vi "TTA_MATLAB_RxOutputPowerTest.vi"(0 "Sub-Function Name":string, 1 "Instrument Cluster In":T2, 5 "Test Group":string, 11 "error in":errorcluster) -> (4 "RxOutput\nPower Results":T1(array[cluster]), 6 "SubTestSuccess":dbl[](array[numeric]), 12 "Instrument Cluster Out":T2, 15 "error out":errorcluster)   [LabVIEW 2016]
uses:
  TTA_Controls/TTA_Control_Complete_Settings_Cluster.ctl
  TTA_Controls/TTA_Control_Instrument_Cluster.ctl
  TTA_Globals/TTA_Global_Complete_Settings.vi
panel:
  out "Channel":string
  out "Rx":string
  out "Test Status":string
  in  "Complete Settings Cluster":T3
  out "RFICs":i32[](array[numeric])
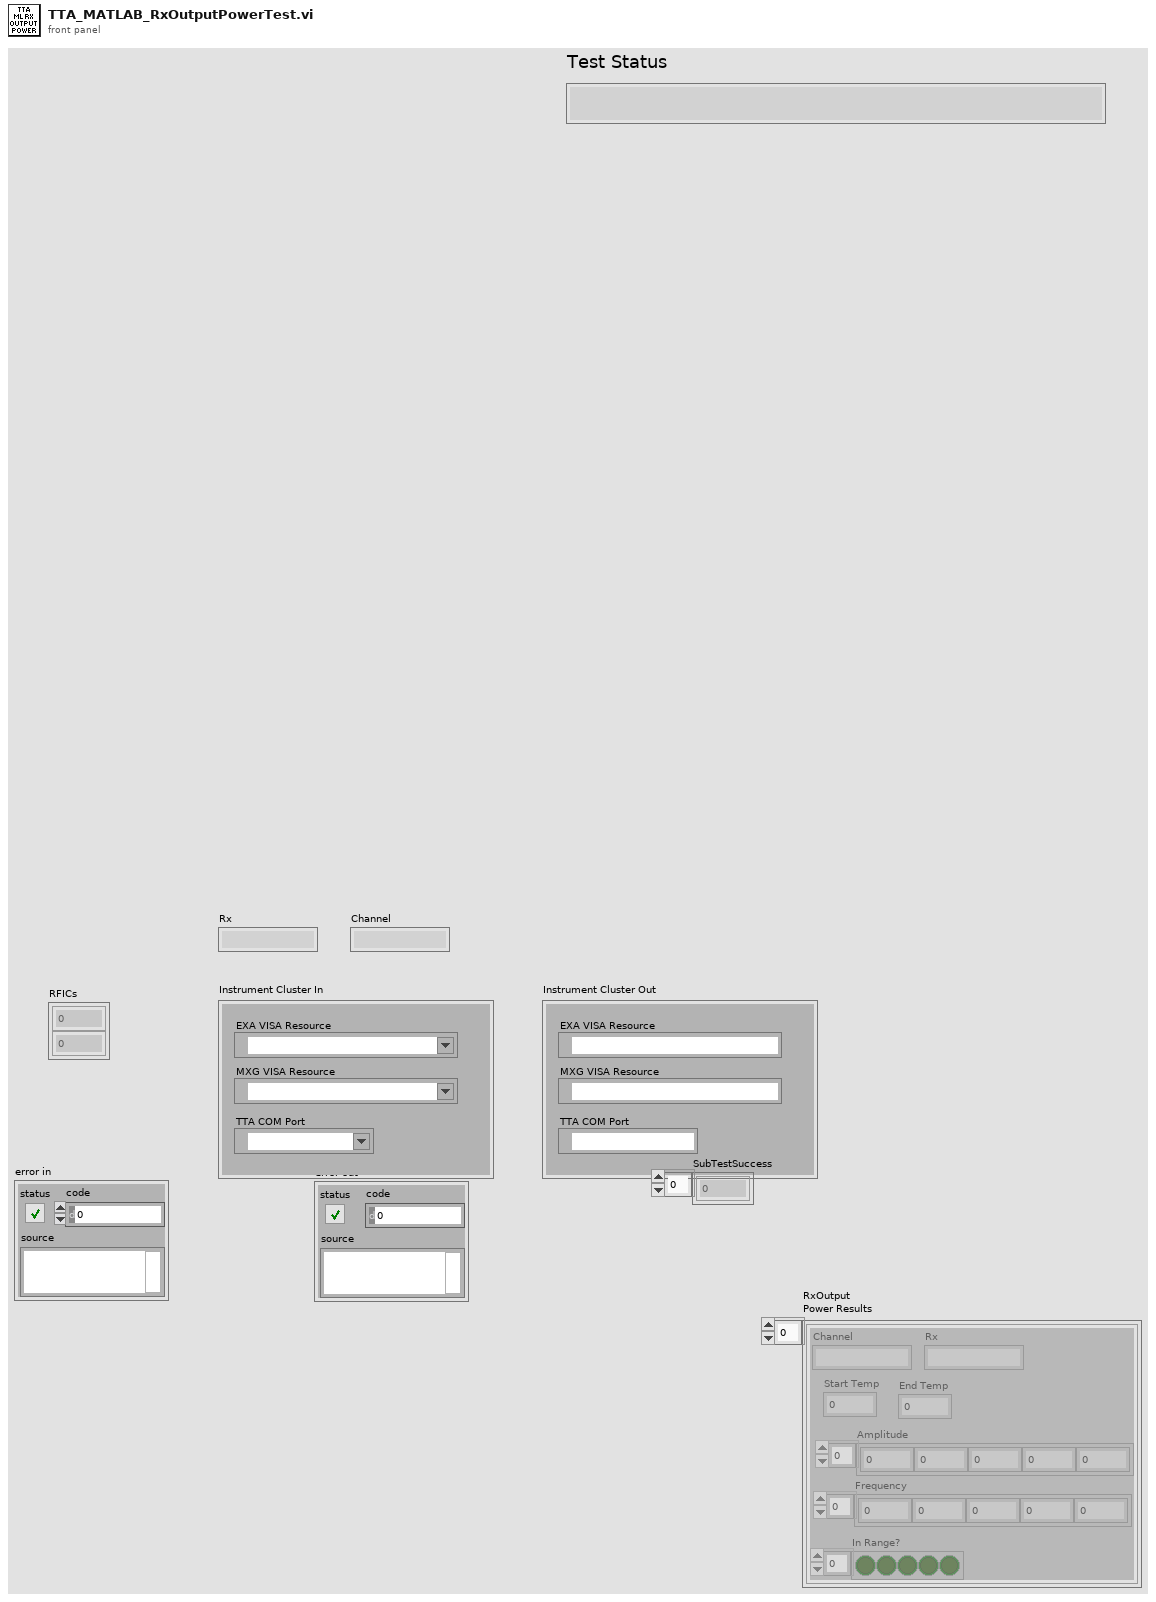
[diagram p1: front panel]
types:
  T1 = cluster{"Channel":string, "Rx":string, "Start Temp":dbl, "End Temp":dbl, "Amplitude":dbl[], "Frequency":dbl[], "In Range?":bool[]}[]
  T2 = typedef "TTA_Control_Instrument_Cluster.ctl" = cluster{"EXA VISA Resource":refnum<visa-resource-name>, "MXG VISA Resource":refnum<visa-resource-name>, "TTA COM Port":refnum<visa-resource-name>}
  T3 = typedef "TTA_Control_Complete_Settings_Cluster.ctl" = cluster{"Brief Cluster":cluster{"STM Firmware File":string, "STM Firmware Address":string, "Required SW Version":string, "Template Used":string}, "Instrument Setting Cluster":cluster{"BDSFreq":dbl, "BDS Amp":dbl, "TxRFCal_Freq":dbl, "TxRFCal_Amp":dbl, "RxRFCal_Freq":dbl, "RxRFCal_Freq":dbl, "TxIF_Freq":dbl, "TxIF_Amp":dbl, "Tx_Output_Power_Signal_Freq":dbl, "Tx_ACPR_Signal_Freq":dbl, "Rx_RF_Freq":dbl, "Rx_RF_Amp":dbl, "Rx_Output_Power_Signal_Freq":dbl, "Rx_Output_Power_Sense_Freq":dbl}, "PAL Calibration\nInputs Cluster":cluster{"Amplitude Range\nMax(dBm)":dbl, "Amplitude Range\nMin(dBm)":dbl, "Amplitude Least\nCriteria (dBm)":dbl, "Frequency 1":dbl, "Frequency 2":dbl, "Frequency 3":dbl, "CAL Amplitude\nDecrement (dB)":dbl, "CAL Amplitude\nIncrement(dB)":dbl, "DownloadFile":string}, "TxOffset Cal Cluster":cluster{"Tx1 Offset (dB)":dbl, "Tx2 Offset (dB)":dbl, "Tx3 Offset (dB)":dbl, "Tx4 Offset (dB)":dbl, "Total RF Tx Loss (dB)":dbl}, "RxOffset Cal Cluster":cluster{"Rx1 Offset (dB)":dbl, "Rx2 Offset (dB)":dbl, "Rx3 Offset (dB)":dbl, "Rx4 Offset (dB)":dbl, "Total RF Rx Loss (dB)":dbl}, "TX Output Power Settings Cluster":cluster{"Frequency Sweep (MHz)":dbl[], "Sig Gen \nPower (dBm)":dbl, "Span (kHz)":dbl, "RBW (Hz)":dbl, "Ref Level (dBm)":dbl, "Low Power \nLimit":dbl, "High Power \nLimit":dbl, "DigAtt Max":dbl, "DigAtt Min":dbl}, "Tx ACPR Settings Cluster":cluster{"ACPR Filename":string, "Sampling Rate":dbl, "Power (dBm)":dbl, "IF Frequency Sweep (MHz)":dbl[], "State Name":string, "Mechanical\nAttenuation":dbl, "RefLevel Offset":dbl, "Amplitude Range\nMax (dBm)":dbl, "Amplitude Range\nMin (dBm)":dbl, "Cal Amp \nIncrement (dB)":dbl, "Cal Amp\nDecrement (dB)":dbl}, "Power Cal Cluster":cluster{"Power List (dBm)":dbl[], "Frequency (MHz)":dbl[], "Cal Decrement (dB)":dbl, "Cal Increment (dB)":dbl}, "Rx Received Power Settings Cluster":cluster{"Frequency Sweep (MHz)":dbl[], "Power (dBm)":dbl, "Span (kHz)":dbl, "RBW (Hz)":dbl, "Ref Level":dbl, "Low Power \nLimit (dBm)":dbl, "High Power\nLimit (dBm)":dbl}, "Tx Output Power Criteria Cluster":cluster{"CH1-TX1 \nMin":dbl, "CH1-TX1\nMax":dbl, "CH1-TXx3\nMin ":dbl, "CH1-TXx3\nMax":dbl, "CH2-TX1\nMin":dbl, "CH2-TX1\nMax":dbl, "CH2-TXx3\nMin":dbl, "CH2-TXx3\nMax":dbl}, "Tx ACPR Criteria Cluster":cluster{"Min Inband":dbl, "Max Close Outband":dbl, "Max Far Outband":dbl}, "Rx Output Power Criteria Cluster":cluster{"CH1-RX1 \nMin":dbl, "CH1-RX1 \nMax":dbl, "CH1-RXx3 \nMin":dbl, "CH1-RXx3\nMax":dbl, "CH2-RX1\nMin":dbl, "CH2-RX1\nMax":dbl, "CH2-RXx3\nMin":dbl, "CH2-RXx3\nMax":dbl}}
  T4 = cluster{"BDSFreq":dbl, "BDS Amp":dbl, "TxRFCal_Freq":dbl, "TxRFCal_Amp":dbl, "RxRFCal_Freq":dbl, "RxRFCal_Freq":dbl, "TxIF_Freq":dbl, "TxIF_Amp":dbl, "Tx_Output_Power_Signal_Freq":dbl, "Tx_ACPR_Signal_Freq":dbl, "Rx_RF_Freq":dbl, "Rx_RF_Amp":dbl, "Rx_Output_Power_Signal_Freq":dbl, "Rx_Output_Power_Sense_Freq":dbl}
  T5 = cluster{"Frequency Sweep (MHz)":dbl[], "Power (dBm)":dbl, "Span (kHz)":dbl, "RBW (Hz)":dbl, "Ref Level":dbl, "Low Power \nLimit (dBm)":dbl, "High Power\nLimit (dBm)":dbl}
  T6 = cluster{"Channel":string, "Rx":string, "Start Temp":dbl, "End Temp":dbl, "Amplitude":dbl[], "Frequency":dbl[], "In Range?":bool[]}
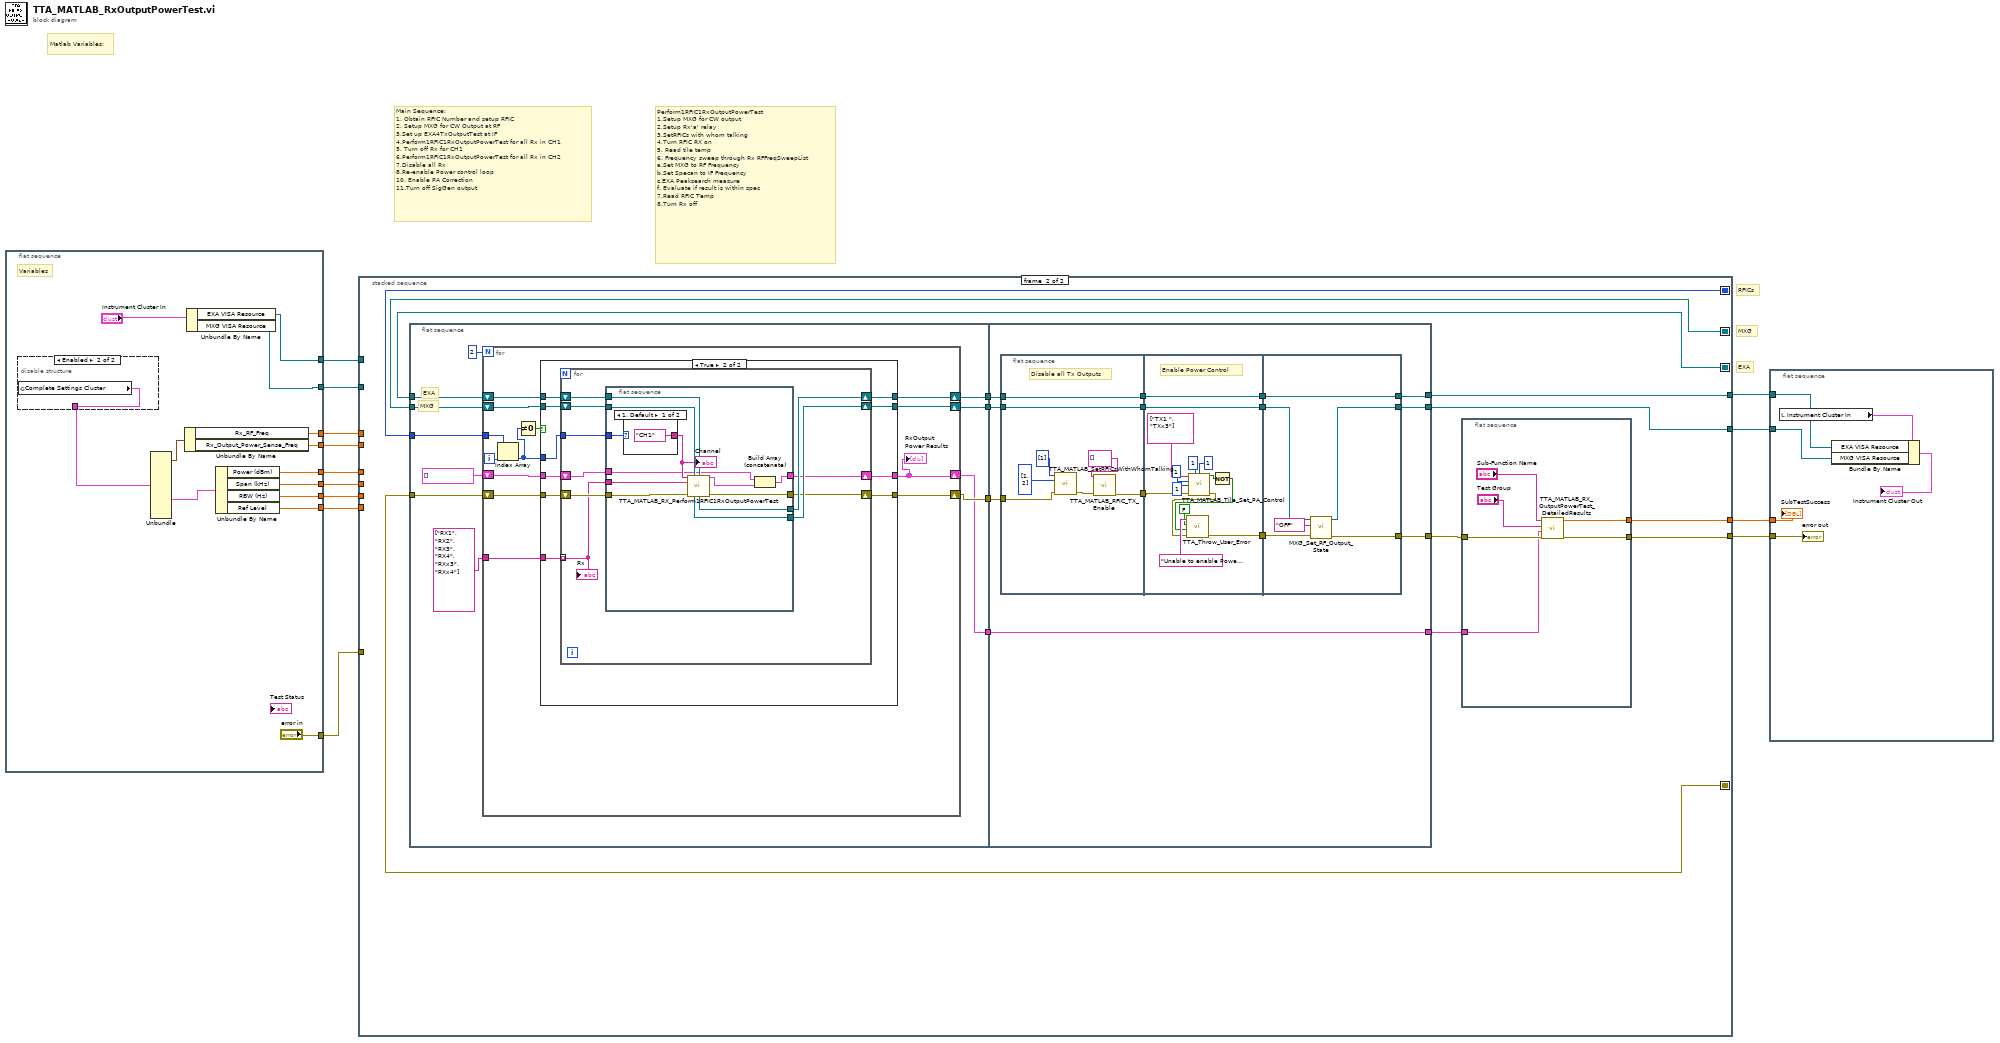
[diagram p0: block diagram]
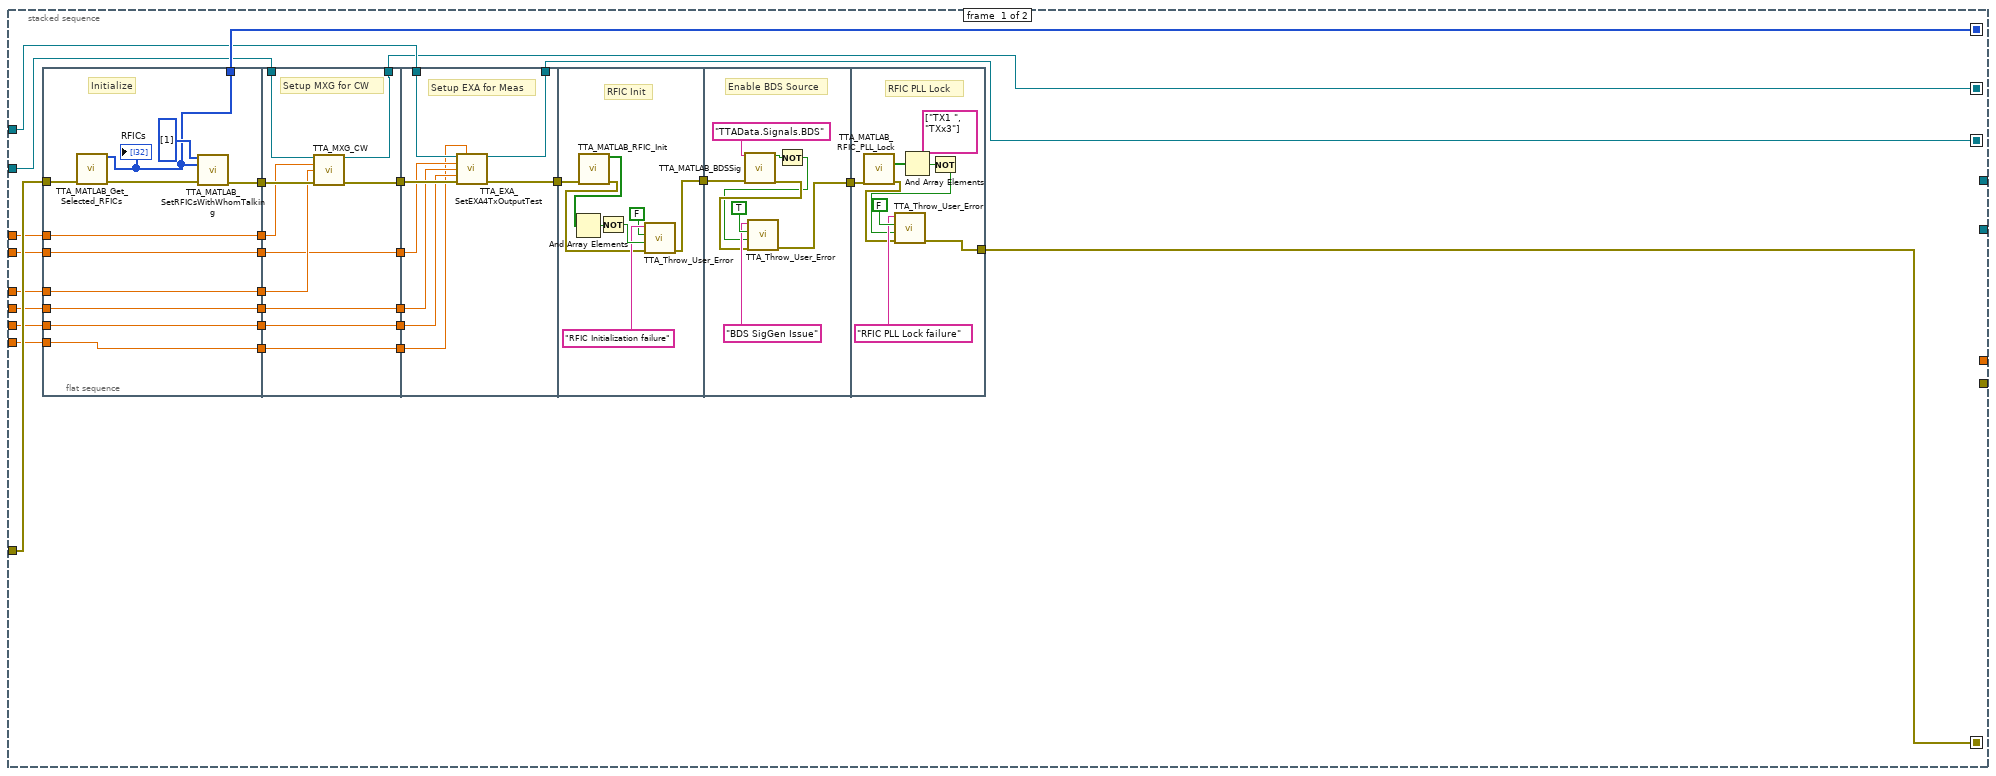
[diagram p2: hidden frame]
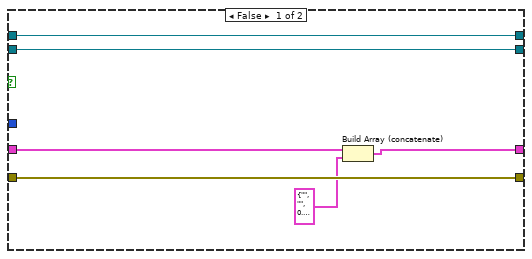
[diagram p3: hidden frame]
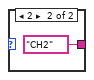
[diagram p4: hidden frame]
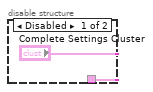
[diagram p5: hidden frame]
diagram:
  # "RFICs"
  # "EXA"
  # "MXG"
  # "Matlab Variables:"
  # "Main Sequence:\n1. Obtain RFIC Number and setup RFIC\n2. Setup MXG for CW Output at RF\n3.Set up EXA4TxOutputTest at IF\n4.Perform1RFIC1RxOutputPowerTest for all Rx in CH1\n5. Turn off Rx for CH1\n6.Perform1RFIC1RxOutputPowerTest for all Rx in CH2\n7.Disable all Rx\n8.Re-enable Power control loop\n10. Enable PA Correction\n11.Turn off SigGen output"
  # "Perform1RFIC1RxOutputPowerTest\n1.Setup MXG for CW output\n2.Setup Rx'a' relay\n3.SetRFICs with whom talking\n4.Turn RFIC RX on\n5. Read tile temp\n6. Frequency sweep through Rx RFFreqSweepList\na.Set MXG to RF Frequency\nb.Set Specan to IF Frequency\nc.EXA Peaksearch measure\nf. Evaluate if result is within spec\n7.Read RFIC Temp\n8.Turn Rx off"
  n1 = flat-sequence {
    tunnel: ["error in"] -> w13
    tunnel: [w23] -> w12
    tunnel: [w22] -> w11
    tunnel: [w19] -> w7
    tunnel: [w18] -> w6
    tunnel: [w17] -> w5
    tunnel: [w16] -> w4
    tunnel: [w15] -> w3
    tunnel: [w14] -> w2
    frame #0 {
      # "Variables"
      n2 = disable-structure shown="Enabled" {
        disable-tunnel: ["Complete Settings Cluster" w28] -> w26
        frame Disabled {
        }
        frame Enabled {
          n3 = global read "TTA_Global_Complete_Settings.vi" "Complete Settings Cluster"() -> (w28:T3)
        }
      }
      n4 = Unbundle(w26) -> ("Instrument Setting Cluster"=w20:T4, "Rx Received Power Settings Cluster"=w21:T5)  [unwired: 10 out]
      n5 = Unbundle By Name(w20) -> ("Rx_RF_Freq"=w19:dbl, "Rx_Output_Power_Sense_Freq"=w17:dbl)
      n6 = Unbundle By Name("Instrument Cluster In") -> ("EXA VISA Resource"=w23:refnum<visa-resource-name>, "MXG VISA Resource"=w22:refnum<visa-resource-name>)
      n7 = Unbundle By Name(w21) -> ("Power (dBm)"=w18:dbl, "Span (kHz)"=w16:dbl, "RBW (Hz)"=w15:dbl, "Ref Level"=w14:dbl)
    }
  }
  n8 = stacked-sequence {
    seq-local: [w55 _] -> [_ w123]
    seq-local: [w31 _] -> [_ w121]
    seq-local: [w29 _] -> [_ w122]
    seq-local: [w30 _] -> [_ w120]
    tunnel: w13 -> [w56 _]
    tunnel: w12 -> [w44 _]
    tunnel: w11 -> [w51 _]
    tunnel: [_ w111] -> w10
    tunnel: [_ w116] -> w9
    tunnel: [_ w115] -> w8
    tunnel: w7 -> [w50 _]
    tunnel: w6 -> [w48 _]
    tunnel: w5 -> [w43 _]
    tunnel: w4 -> [w40 _]
    tunnel: w3 -> [w39 _]
    tunnel: w2 -> [w38 _]
    tunnel: [_ w110] -> w1
    frame #0 {
      n9 = flat-sequence {
        tunnel: w56 -> [w65]
        tunnel: [w64] -> w55
        tunnel: [w63] -> w54
        tunnel: w50 -> [w62]
        tunnel: [w62] -> w49
        tunnel: w48 -> [w61]
        tunnel: [w61] -> w47
        tunnel: w43 -> [w60]
        tunnel: [w60] -> w41
        tunnel: w40 -> [w59]
        tunnel: w39 -> [w58]
        tunnel: w38 -> [w57]
        tunnel: [w59] -> w36
        tunnel: [w58] -> w34
        tunnel: [w57] -> w32
        tunnel: w54 -> [w76]
        tunnel: [w73] -> w46
        tunnel: w51 -> [w77]
        tunnel: w49 -> [w75]
        tunnel: w47 -> [w74]
        tunnel: [w72] -> w42
        tunnel: w41 -> [w72]
        tunnel: [w71] -> w37
        tunnel: w36 -> [w71]
        tunnel: [w70] -> w35
        tunnel: w34 -> [w70]
        tunnel: [w69] -> w33
        tunnel: w32 -> [w69]
        tunnel: [w68] -> w30
        tunnel: w46 -> [w85]
        tunnel: [w78] -> w45
        tunnel: w44 -> [w84]
        tunnel: w42 -> [w83]
        tunnel: w37 -> [w82]
        tunnel: w35 -> [w81]
        tunnel: w33 -> [w80]
        tunnel: [w79] -> w29
        tunnel: w45 -> [w88]
        tunnel: [w86] -> w53
        tunnel: w53 -> [w97]
        tunnel: [w95] -> w52
        tunnel: w52 -> [w104]
        tunnel: [w102] -> w31
        frame #0 {
          # "Initialize"
          n10 = call "TTA_MATLAB_Get_Selected_RFICs.vi"("error in"=w65) -> ("RFICs"=w64:i32[], "error out"=w66:errorcluster)  [unwired: 13 in]
          "RFICs" <- w64
          n11 = call "TTA_MATLAB_SetRFICsWithWhomTalking.vi"("Panel Array"=i32[] [1], "RFIC Array"=w64, "error in"=w66) -> ("error out"=w63:errorcluster)  [unwired: 12 in]
        }
        frame #1 {
          # "Setup MXG for CW"
          n12 = call "TTA_MXG_CW.vi"("VISA resource In"=w77, "Frequency (MHz)"=w75, "Output Power\nLevel (dBm)"=w74, "error in"=w76) -> ("VISA resource Out"=w68:refnum<visa-resource-name>, "error out"=w73:errorcluster)  [unwired: 10 in]
        }
        frame #2 {
          # "Setup EXA for Meas"
          n13 = call "TTA_EXA_SetEXA4TxOutputTest.vi"("VISA resource In"=w84, "Reference Level (dBm)"=w80, "Frequency (MHz)"=w83, "Span (kHz)"=w82, "RBW (Hz)"=w81, "error in"=w85) -> ("VISA resource Out"=w79:refnum<visa-resource-name>, "error out"=w78:errorcluster)  [unwired: 8 in]
        }
        frame #3 {
          # "RFIC Init"
          n14 = call "TTA_MATLAB_RFIC_Init.vi"("error in"=w88) -> ("SuccessComm"=w93:bool[], "error out"=w87:errorcluster)  [unwired: 13 in]
          n15 = And Array Elements(Boolean array=w93) -> (logical AND=w92:bool)
          n16 = Not(x=w92) -> (.not. x?=w91:bool)
          n17 = call "TTA_Throw_User_Error.vi"("error in"=w87, "Error?"=w91, "Stop Execution on Fail"=FALSE, "Error Message"="RFIC Initialization failure") -> ("error out"=w86:errorcluster)  [unwired: 7 in]
        }
        frame #4 {
          # "Enable BDS Source"
          n18 = call "TTA_MATLAB_BDSSig.vi"("Signal Settings"="TTAData.Signals.BDS", "error in"=w97) -> ("Success"=w98:bool, "error out"=w96:errorcluster)  [unwired: 12 in]
          n19 = Not(x=w98) -> (.not. x?=w94:bool)
          n20 = call "TTA_Throw_User_Error.vi"("error in"=w96, "Error?"=w94, "Stop Execution on Fail"=TRUE, "Error Message"="BDS SigGen Issue") -> ("error out"=w95:errorcluster)  [unwired: 7 in]
        }
        frame #5 {
          (unwired) string[] ["TX1 ", "TXx3"] ("Channels")
          # "RFIC PLL Lock"
          n21 = call "TTA_MATLAB_RFIC_PLL_Lock.vi"("error in"=w104) -> ("SuccessComm"=w109:bool[], "error out"=w103:errorcluster)  [unwired: 11 in, 2 out]
          n22 = And Array Elements(Boolean array=w109) -> (logical AND=w106:bool)
          n23 = Not(x=w106) -> (.not. x?=w105:bool)
          n24 = call "TTA_Throw_User_Error.vi"("error in"=w103, "Error?"=w105, "Stop Execution on Fail"=FALSE, "Error Message"="RFIC PLL Lock failure") -> ("error out"=w102:errorcluster)  [unwired: 7 in]
        }
      }
    }
    frame #1 {
      n25 = flat-sequence {
        tunnel: w123 -> [w140]
        tunnel: w122 -> [w139]
        tunnel: w120 -> [w138]
        tunnel: w121 -> [w137]
        tunnel: [w136] -> w119
        tunnel: [w135] -> w118
        tunnel: [w134] -> w117
        tunnel: [w130] -> w113
        tunnel: w119 -> [w206]
        tunnel: w118 -> [w205]
        tunnel: w117 -> [w204]
        tunnel: [w197] -> w114
        tunnel: [w196] -> w116
        tunnel: [w195] -> w115
        tunnel: w113 -> [w194]
        tunnel: [w194] -> w112
        frame #0 {
          # "EXA"
          # "MXG"
          n26 = for {
            N: 2 -> [_]
            tunnel: w140 -> [w145]
            shift-right: [w151] -> w135
            shift-left: w139 -> [w150]
            shift-right: [w148] -> w134
            shift-left: w138 -> [w149]
            shift-right: [w147] -> w136
            shift-left: w137 -> [w153]
            tunnel: string[] ["RX1", "RX2", "RX3", "RX4", "RXx3", "RXx4"] -> [w152]
            shift-right: [w141] -> w130
            shift-left: T1 [] -> [w146]
            i -> [w144]
            n27 = Index Array(array=w145, index=w144) -> (element=w142:i32)
            n28 = Not Equal To 0?(x=w142) -> (x != 0?=w143:bool)
            n29 = case shown="True" w143 {
              tunnel: w153 -> [w159 w169]
              tunnel: w152 -> [_ w168]
              tunnel: [w155 w167] -> w151
              tunnel: w150 -> [w155 w166]
              tunnel: w149 -> [w154 w165]
              tunnel: [w154 w164] -> w148
              tunnel: [w159 w163] -> w147
              tunnel: w146 -> [w157 w162]
              tunnel: [w156 w161] -> w141
              tunnel: w142 -> [_ w160]
              frame False {
                n30 = Build Array (concatenate)(w157, T6 {"Channel"="", "Rx"="", "Start Temp"=0.0, "End Temp"=0.0, "Amplitude"=[], "Frequency"=[], "In Range?"=[]} ("Output Power\nResults")) -> (w156:T1)
              }
              frame True {
                n31 = for {
                  tunnel: w160 -> [w179]
                  tunnel: w168 -> [w177] mode=indexing
                  shift-right: [w176] -> w167
                  shift-left: w166 -> [w175]
                  shift-right: [w174] -> w164
                  shift-left: w165 -> [w173]
                  shift-right: [w172] -> w163
                  shift-left: w169 -> [w178]
                  shift-right: [w171] -> w161
                  shift-left: w162 -> [w170]
                  n32 = flat-sequence {
                    tunnel: w179 -> [w191]
                    tunnel: w175 -> [w190]
                    tunnel: w173 -> [w189]
                    tunnel: w178 -> [w188]
                    tunnel: w177 -> [w180]
                    tunnel: [w186] -> w176
                    tunnel: [w185] -> w174
                    tunnel: [w184] -> w172
                    tunnel: [w182] -> w171
                    tunnel: w170 -> [w181]
                    frame #0 {
                      n33 = case shown="1, Default" w191 {
                        tunnel: ["CH1" ("Channel") "CH2" ("Channel")] -> w187
                        frame 1, Default {
                        }
                        frame 2 {
                        }
                      }
                      "Channel" <- w187
                      n34 = call "TTA_MATLAB_RX_Perform1RFIC1RxOutputPowerTest.vi"("Channel"=w187, "MXG VISA Resource In"=w189, "EXA VISA Resource"=w190, "Rx"=w180, "error in"=w188) -> ("Output Power\nResults"=w183:T6, "MXG VISA Resource Out"=w185:refnum<visa-resource-name>, "EXA VISA Resource Out"=w186:refnum<visa-resource-name>, "error out"=w184:errorcluster)  [unwired: 7 in]
                      n35 = Build Array (concatenate)(w181, w183) -> (w182:T1)
                    }
                  }
                  "Rx" <- w177
                }
              }
            }
            "RxOutput\nPower Results" <- w141
          }
        }
        frame #1 {
          n36 = flat-sequence {
            tunnel: w206 -> [w212]
            tunnel: w205 -> [w208]
            tunnel: w204 -> [w207]
            tunnel: [w209] -> w203
            tunnel: [w208] -> w202
            tunnel: [w207] -> w201
            tunnel: w203 -> [w217]
            tunnel: w202 -> [w228]
            tunnel: w201 -> [w227]
            tunnel: [w228] -> w200
            tunnel: [w227] -> w199
            tunnel: [w215] -> w198
            tunnel: [w231] -> w196
            tunnel: [w234] -> w195
            tunnel: w200 -> [w234]
            tunnel: w199 -> [w232]
            tunnel: w198 -> [w233]
            tunnel: [w229] -> w197
            frame #0 {
              # "Disable all Tx Outputs"
              n37 = call "TTA_MATLAB_SetRFICsWithWhomTalking.vi"("Panel Array"=i32[] [1], "RFIC Array"=i32[] [1, 2], "error in"=w212) -> ("error out"=w210:errorcluster)  [unwired: 12 in]
              n38 = call "TTA_MATLAB_RFIC_TX_Enable.vi"("Channels"=string[] [], "error in"=w210) -> ("error out"=w209:errorcluster)  [unwired: 12 in, 1 out]
            }
            frame #1 {
              # "Enable Power Control"
              n39 = call "TTA_MATLAB_Tile_Set_PA_Control.vi"("Channels"=string[] ["TX1 ", "TXx3"], "OutPower"=1, "InPower"=1, "Temp"=1, "Current"=1, "error in"=w217) -> ("Success"=w220:bool, "error out"=w218:errorcluster)  [unwired: 6 in, 2 out]
              n40 = Not(x=w220) -> (.not. x?=w219:bool)
              n41 = call "TTA_Throw_User_Error.vi"("error in"=w218, "Error?"=w219, "Stop Execution on Fail"=FALSE, "Error Message"="Unable to enable Power Loop") -> ("error out"=w215:errorcluster)  [unwired: 7 in]
            }
            frame #2 {
              n42 = call "MXG_Set_RF_Output_State.vi"("error in"=w233, "RF Output State"="OFF", "VISA resource name"=w232) -> ("error out"=w229:errorcluster, "VISA resource name"=w231:refnum<visa-resource-name>)  [unwired: 7 in]
            }
          }
        }
      }
      n43 = flat-sequence {
        tunnel: w114 -> [w129]
        tunnel: w112 -> [w128]
        tunnel: [w125] -> w111
        tunnel: [w124] -> w110
        frame #0 {
          n44 = call "TTA_MATLAB_RX_OutputPowerTest_DetailedResults.vi"("error in"=w129, "RxOutput\nPower Results"=w128, "TestGroup"="Test Group", "SubTest"="Sub-Function Name") -> ("error out"=w125:errorcluster, "SubTestSuccess"=w124:dbl[])  [unwired: 6 in]
        }
      }
    }
  }
  n45 = flat-sequence {
    tunnel: w10 -> [w240]
    tunnel: w9 -> [w237]
    tunnel: w8 -> [w238]
    tunnel: w1 -> [w235]
    frame #0 {
      n46 = local read "Instrument Cluster In"() -> (w236:T2)
      n47 = Bundle By Name(cluster=w236, "EXA VISA Resource"=w238, "MXG VISA Resource"=w237) -> (→"Instrument Cluster Out":T2)
      "error out" <- w240
      "SubTestSuccess" <- w235
    }
  }
